vi "lv create channel.vi"(7 "stream":i32, 8 "error in (no error)":errorcluster, 11 "name":string) -> (0 "error out":errorcluster, 3 "channel handle":i32)   [LabVIEW 2026]
uses:
  bin/nominalClient_64.dll
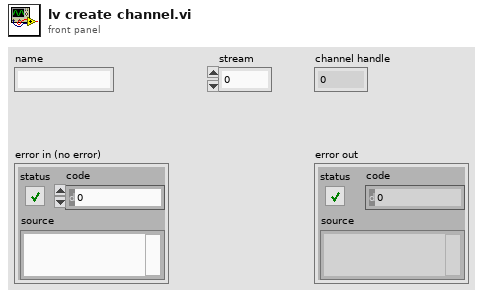
[diagram p1: front panel]
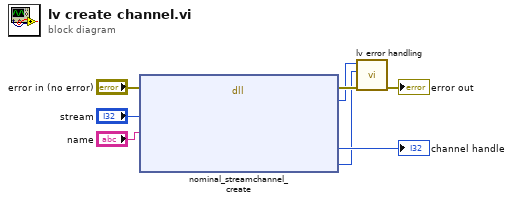
[diagram p0: block diagram]
diagram:
  n1 = dll-call lib="C:/sw/nominal-c/bin/nominalClient_64.dll" fn="nominal_streamchannel_create"(error in="error in (no error)", "stream"="stream", "name"="name") -> (error out=w4:errorcluster, "return type"=w3:i32, "channel handle"=→"channel handle":i32, "errorout"=w2:i32)  [unwired: 6 in, 1 out]
  n2 = call "lv error handling.vi"("error in"=w4, "error handle"=w2, "return code"=w3) -> ("error out"=→"error out":errorcluster)  [unwired: 8 in]
